vi "Or.vi"(0 "A":bool, 5 "B":bool, 7 "STOP":bool, 11 "Error in":errorcluster) -> (8 "Or":bool, 15 "Error out":errorcluster)   [LabVIEW 2020, in "Subpanel access.lvlib"]
uses:
  Subpanel access.lvlib
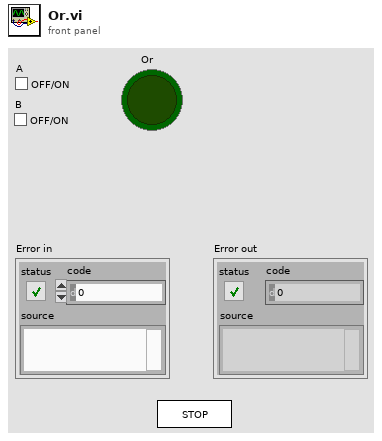
[diagram p1: front panel]
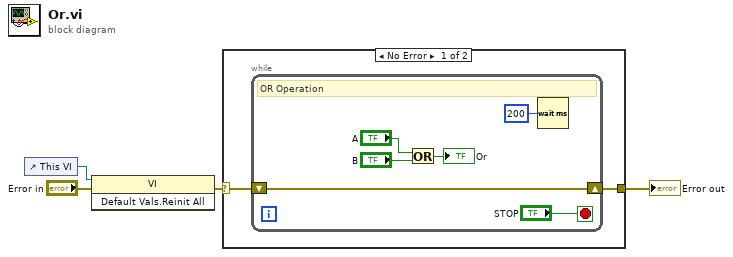
[diagram p0: block diagram]
diagram:
  n1 = control-ref of="This VI"() -> (w1:refnum<vi>)
  n2 = invoke class="VI" method="Default Vals.Reinit All"(reference=w1, error in="Error in") -> (error out=w2:errorcluster)  [unwired: 1 in, 2 out]
  n3 = case shown="No Error" w2 {
    selector: w2 -> [w5 w13]
    tunnel: [w6 w13] -> w4
    frame No Error {
      n4 = while {
        shift-right: [w12] -> w6
        shift-left: w5 -> [w12]
        stop <- "STOP" stop-if-true
        # "OR Operation"
        n5 = Or(x="A", y="B") -> (x .or. y?=→"Or":bool)
        n6 = Wait (ms)(milliseconds to wait=u32 200) -> ()  [unwired: 1 out]
      }
    }
    frame Error {
    }
  }
  "Error out" <- w4
